vi "server.vi"() -> ()   [LabVIEW 2013]
uses:
  global_var.vi
panel:
  out "string to be\nsend":string
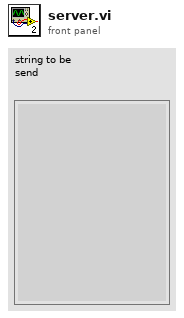
[diagram p1: front panel]
types:
  T1 = enum16{"Standard", "Buffered", "CRLF", "Immediate"}
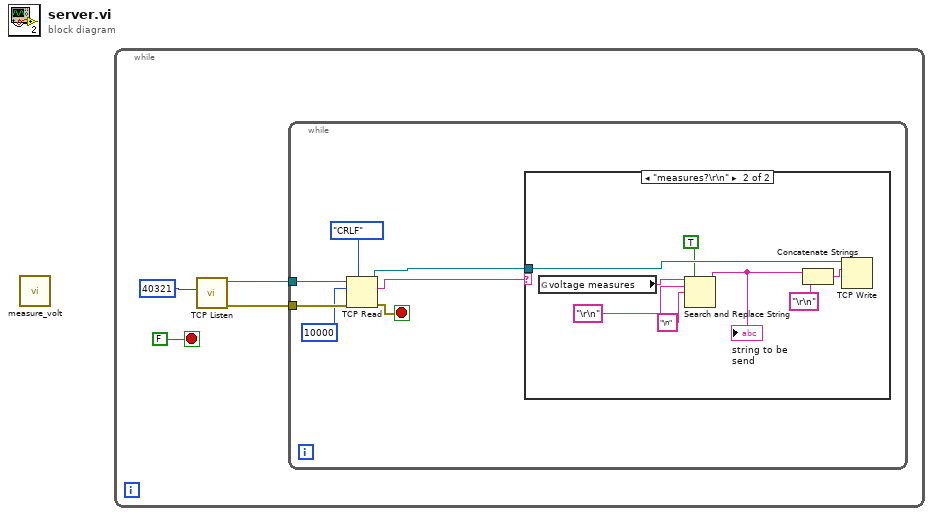
[diagram p0: block diagram]
diagram:
  n1 = call "measure_volt.vi"() -> ()  [unwired: 11 in]
  n2 = while {
    stop <- FALSE stop-if-true
    n3 = call <vilib>:"TCP Listen.vi"("port"=u16 40321) -> ("error out"=w2:errorcluster, "connection ID"=w4:refnum<k5>)  [unwired: 6 in, 3 out]
    n4 = while {
      tunnel: w4 -> [w11]
      tunnel: w2 -> [w6]
      stop <- w7 stop-if-true
      n5 = TCP Read(connection ID=w11, bytes to read=10000, error in (no error)=w6, 7:T1."CRLF" ("mode (standard)")) -> (connection ID out=w8:refnum<k5>, data out=w9:string, error out=w7:errorcluster)  [unwired: 1 in]
      n6 = case shown="\"measures?\\r\\n\"" w9 {
        tunnel: w8 -> [_ w19]
        frame "False", Default {
        }
        frame "measures?\r\n" {
          n7 = global read "global_var.vi" "voltage measures"() -> (w15:string)
          n8 = Search and Replace String(replace all?=TRUE ("replace all? (F)"), input string=w15, search string="\r\n", replace string="\n" ("replace string (\"\")")) -> (result string=w16:string)  [unwired: 4 in, 3 out]
          "string to be\nsend" <- w16
          n9 = Concatenate Strings(w16, "\r\n" ("string")) -> (w17:string)
          n10 = TCP Write(connection ID=w19, data in=w17) -> ()  [unwired: 2 in, 3 out]
        }
      }
    }
  }
